vi "Array of Variants to Cluster Variant.vi"(8 "error in (no error)":errorcluster, 11 "[Variant]":variant[](array[variant])) -> (0 "error out":errorcluster, 3 "Cluster Variant":variant)   [LabVIEW 2018, in "Potentiostat Galvanostat.lvclass"]
uses:
  Potentiostat Galvanostat.lvclass
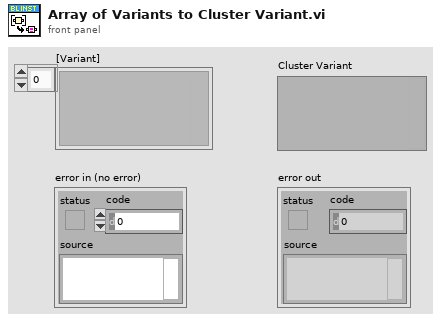
[diagram p1: front panel]
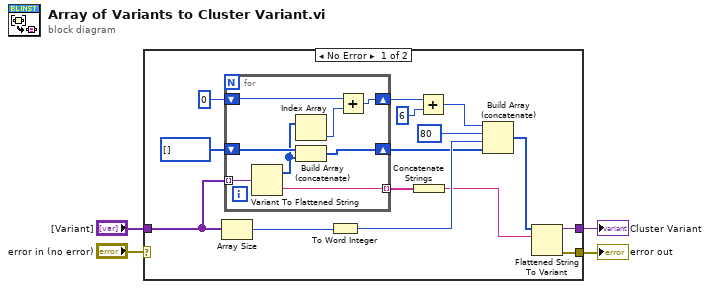
[diagram p0: block diagram]
diagram:
  n1 = case shown="No Error" "error in (no error)" {
    selector: "error in (no error)" -> [_ w28]
    tunnel: [w10 w28] -> w2
    tunnel: [w9 _] -> w1
    tunnel: "[Variant]" -> [w6 _]
    frame No Error {
      n2 = Array Size(array=w6) -> (size(s)=w5:i32)
      n3 = for {
        tunnel: w6 -> [w27] mode=indexing
        shift-right: [w20] -> w12
        shift-left: i16[] [] ("type string") -> [w26]
        shift-right: [w22] -> w17
        shift-left: i16 0 -> [w23]
        tunnel: [w21] -> w8 mode=indexing
        n4 = Variant To Flattened String(Variant=w27) -> (data string=w21:string, 1:w25:i16[])
        n5 = Index Array(array=w25) -> (element=w24:i16)  [unwired: 1 in]
        n6 = Build Array (concatenate)(w26, w25) -> (w20:i16[])
        n7 = Add(x=w23, y=w24) -> (x+y=w22:i16)
      }
      n8 = To Word Integer(number=w5) -> (16bit integer=w13:i16)
      n9 = Concatenate Strings(w8) -> (w7:string)
      n10 = Add(x=w17, y=i16 6) -> (x+y=w15:i16)
      n11 = Build Array (concatenate)(w15, i16 80, w13, w12) -> (w11:i16[])
      n12 = Flattened String To Variant(6:w7, 7:w11) -> (0:w10:errorcluster, 3:w9:variant)  [unwired: 1 in]
    }
    frame Error {
    }
  }
  "error out" <- w2
  "Cluster Variant" <- w1
